vi "Hardware - NI 9759-1 (Throttle) Host.vi"() -> ()   [LabVIEW 2015, in "ECS-Host.lvlib"]
uses:
  ECS-Host.lvlib
  Typedefs/MISC/Throttle Mode Request.ctl
  ECS-Shared.lvlib
panel:
  out "FPGAInterfaceError":bool
  in  "ModuleEnable":bool
  out "ModulePresent":bool
  in  "_Throttle Channels":T1(tab)
  in  "_Throttle Settings":T2(tab)
  in  "Init":bool
  in  "PrimaryPsnSwitch":bool
  in  "ModeRequest":T3
  out "SecondaryPsn":sgl
  out "uLimit":bool
  out "PrimaryPsn":sgl
  out "Psn_Fault":bool
  out "u":sgl caption="[]"
  out "AboveLH":bool
  out "uLHc":sgl caption="[]" format="%.2f"
  out "uFc":sgl caption="[]" format="%.2f"
  out "uPID":sgl caption="[]" format="%.2f"
  out "Analog2":sgl caption="[]"
  out "Analog1":sgl caption="[]"
  out "H2Sense":sgl caption="[]"
  out "H1Sense":sgl caption="[]"
  out "H2Fault":bool
  out "H1Fault":bool
  out "Battery":sgl caption="[]" format="%.3f"
  out "Temperature":sgl caption="[]" format="%.3f"
  in  "Ch1Enable":bool
  in  "Ch1Freq":sgl caption="[]" format="%.3f"
  out "ModeStatus":T3
  out "PsnCalDiff_Fault":bool
  out "SecondaryAnalogRange":sgl[](array[numeric]) caption="[]"
  out "uLimitNeg":bool
  out "uLimitPos":bool
  out "PsnCalComplete":bool
  out "uPsnCalNeg":sgl caption="[]"
  out "uPsnCalPos":sgl caption="[]"
  out "PrimaryAnalogRange":sgl[](array[numeric]) caption="[]"
  out "PsnRange_Out":sgl[](array[numeric]) caption="[]"
  in  "Analog2Range":sgl[](array[numeric])=[5.0, 0.0] caption="[]"
  in  "PsnRange_In":sgl[](array[numeric])=[0.0, 100.0] caption="[]"
  in  "Analog1Range":sgl[](array[numeric])=[0.0, 5.0] caption="[]"
  in  "PsnCalDiff_Thresh":sgl=3.0 caption="[]" min=0
  in  "PsnCalOffset":sgl=0.005 caption="[]" min=0
  in  "uPsnCalNeg_Init":sgl=-3.0 caption="[]" max=0
  in  "uPsnCalPos_Init":sgl=3.4 caption="[]" min=0
  in  "PsnCalReturnFromNegDelay":sgl=1.0 caption="[]" min=0
  in  "uPsnCalDec":sgl=-0.2 caption="[]" max=0
  in  "uPsnCalDec_Thresh":sgl=-1.1 caption="[]" max=0
  in  "PsnCalReturnFromPosDelay":sgl=1.0 caption="[]" min=0
  in  "uPsnCalInc_Thresh":sgl=1.1 caption="[]" min=0
  in  "uPsnCalInc":sgl=0.2 caption="[]" min=0
  in  "PsnCalInitDelay":sgl=1.0 caption="[]" min=0
  out "Psn_FaultThreshOut":sgl caption="[]"
  out "MotorResistance_Out":sgl caption="[]"
  out "LHPsn_Out":sgl caption="[]" format="%.3f"
  out "ULH_Out":sgl caption="[]"
  out "US_Out":sgl caption="[]"
  out "ULHLag_Out":sgl caption="[]" format="%.3f"
  out "USLag_Out":sgl caption="[]" format="%.3f"
  out "LHPsnBand_Out":sgl caption="[]"
  out "TDNeg_Out":sgl caption="[]"
  out "TINeg_Out":sgl caption="[]"
  out "KRNeg_Out":sgl caption="[]"
  out "TLead_Out":sgl caption="[]" format="%.3f"
  out "TDPos_Out":sgl caption="[]"
  out "TIPos_Out":sgl caption="[]"
  out "KRPos_Out":sgl caption="[]"
  out "TLag_Out":sgl caption="[]" format="%.3f"
  in  "Psn_FaultThresh":sgl=5.0 caption="[]"
  in  "MotorResistance":sgl=2.4 caption="[]"
  in  "LHPsn":sgl=5.0 caption="[]" format="%.3f"
  in  "ULH":sgl=1.5 caption="[]"
  in  "US":sgl=0.5 caption="[]"
  in  "ULHLag":sgl=0.06 caption="[]" format="%.3f"
  in  "USLag":sgl=0.15 caption="[]" format="%.3f"
  in  "LHPsnBand":sgl=0.2 caption="[]"
  in  "TDNeg":sgl=0.001 caption="[]"
  in  "TINeg":sgl=0.1 caption="[]"
  in  "KRNeg":sgl=1.0 caption="[]"
  in  "TLead":sgl caption="[]" format="%.3f"
  in  "TDPos":sgl=0.01 caption="[]"
  in  "TIPos":sgl=0.15 caption="[]"
  in  "KRPos":sgl=0.5 caption="[]"
  in  "TLag":sgl=0.1 caption="[]" format="%.3f"
  out "Ch2DutyCyc_Des":sgl caption="[]" format="%.3f"
  in  "Ch2Enable":bool
  in  "Ch2Freq":sgl caption="[]" format="%.3f"
  # "Postion Calibration Settings"
  # "Postion Calibration In"
  # "Postion Calibration Out"
  # "Control Calibration Out"
  # "Control Calibration In"
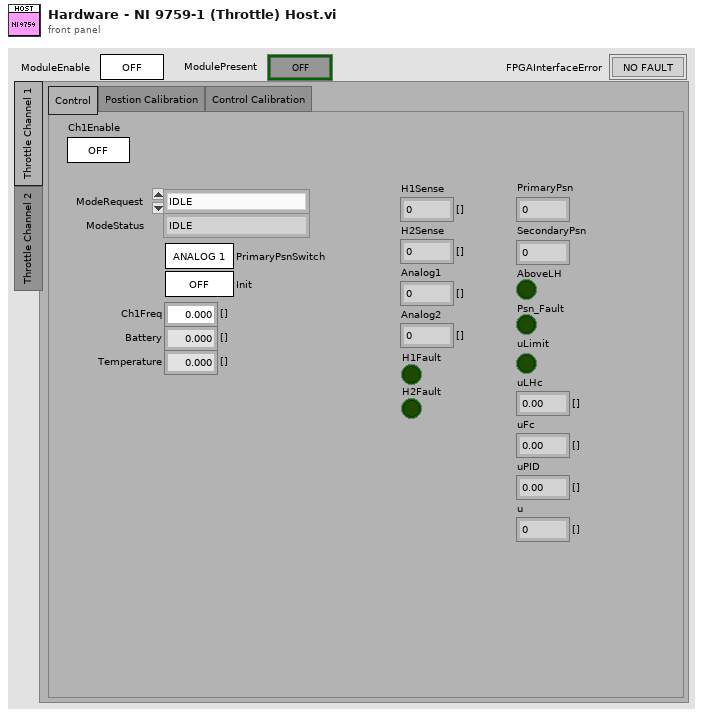
[diagram p1: front panel]
types:
  T1 = enum32{"Throttle Channel 1", "Throttle Channel 2"}
  T2 = enum32{"Control", "Postion Calibration", "Control Calibration"}
  T3 = typedef "ECS-Shared.lvlib/Throttle Mode Request.ctl" = enum32{"IDLE", "POSITION CALIBRATION", "CONTROL CALIBRATION", "CONTROL"}
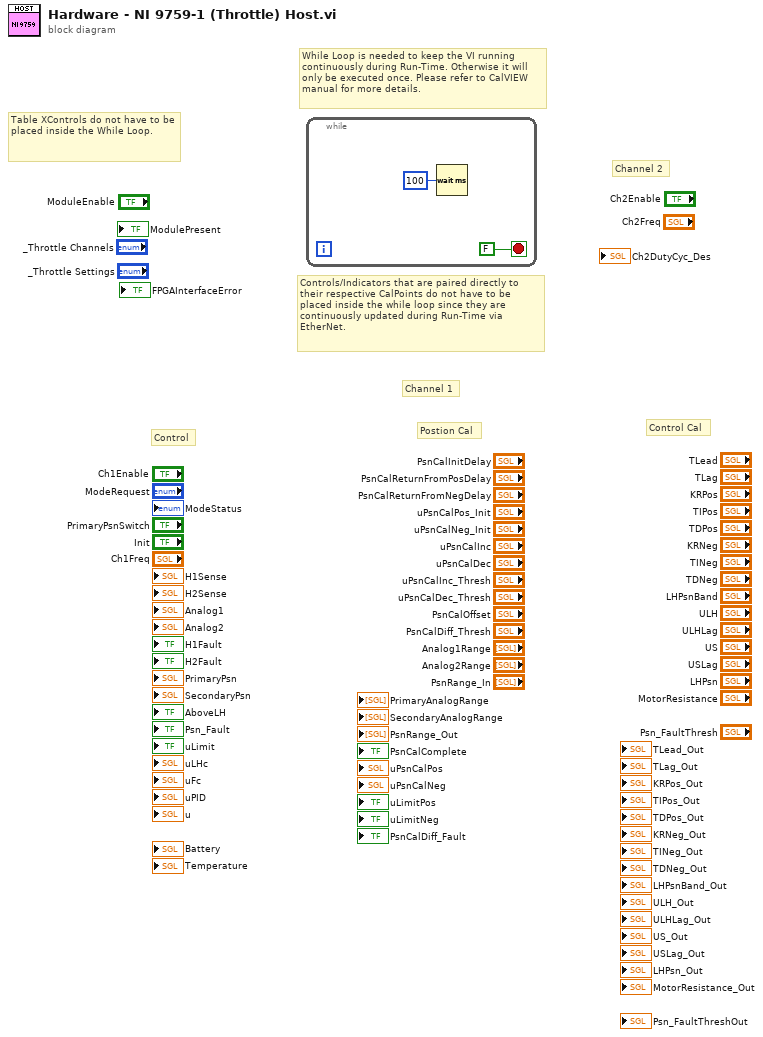
[diagram p0: block diagram]
diagram:
  # "Channel 2"
  # "Channel 1"
  # "Control Cal"
  # "Postion Cal"
  # "Control"
  # "Controls/Indicators that are paired directly to their respective CalPoints do not have to be placed inside the while loop since they are continuously updated during Run-Time via EtherNet."
  # "Table XControls do not have to be placed inside the While Loop."
  # "While Loop is needed to keep the VI running\ncontinuously during Run-Time. Otherwise it will only be executed once. Please refer to CalVIEW manual for more details."
  n1 = while {
    stop <- FALSE stop-if-true
    n2 = Wait (ms)(milliseconds to wait=u32 100) -> ()  [unwired: 1 out]
  }
